vi "Configure System.vi"(8 "error in (no error)":errorcluster, 11 "System Configuration":T1) -> (0 "error out":errorcluster, 3 "dup System Configuration":T1)   [LabVIEW 2024]
doc: "Applies system configurations."
uses:
  Controls/Server/System Configuration.ctl
  Controls/Server/Subsystem Configuration.ctl
  <vilib>/lvdsc/NI_DSC.lvlib
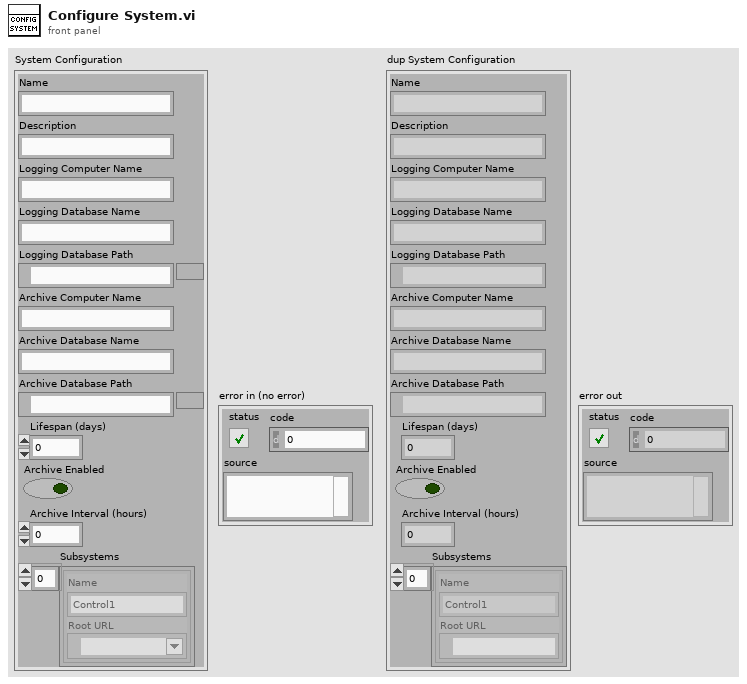
[diagram p1: front panel]
types:
  T1 = typedef "System Configuration.ctl" = cluster{"Name":string, "Description":string, "Logging Computer Name":string, "Logging Database Name":string, "Logging Database Path":path, "Archive Computer Name":string, "Archive Database Name":string, "Archive Database Path":path, "Lifespan (days)":u32, "Archive Enabled":bool, "Archive Interval (hours)":u32, "Subsystems":T2[]}
  T2 = typedef "Subsystem Configuration.ctl" = cluster{"Name":string, "Root URL":refnum<k21>}
  T3 = cluster{"machine":string, "name":string, "path":path}
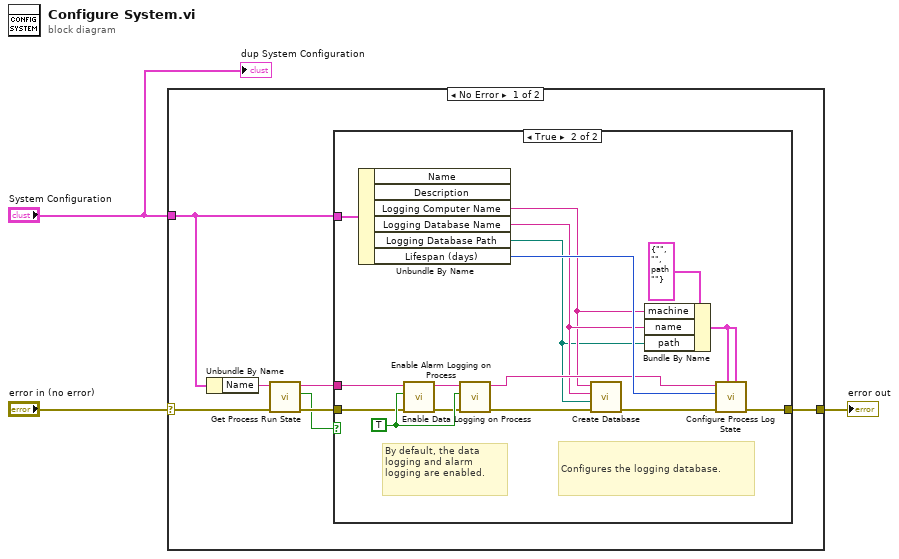
[diagram p0: block diagram]
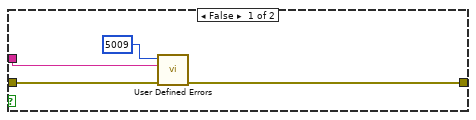
[diagram p2: hidden frame]
diagram:
  n1 = case shown="No Error" "error in (no error)" {
    selector: "error in (no error)" -> [w5 w31]
    tunnel: [w7 w31] -> w3
    tunnel: "System Configuration" -> [w4 _]
    frame No Error {
      n2 = Unbundle By Name(w4) -> ("Name"=w10:string)
      n3 = call <vilib>:"Get Process Run State.vi"("error in (no error)"=w5, "process name"=w10) -> ("error out"=w8:errorcluster, "exists?"=w6:bool, "process name out"=w9:string)  [unwired: 6 in, 1 out]
      n4 = case shown="True" w6 {
        tunnel: w9 -> [w13 w26]
        tunnel: w8 -> [w12 w27]
        tunnel: [w11 w15] -> w7
        tunnel: w4 -> [_ w25]
        frame False {
          n5 = call "User Defined Errors.vi"("error in (no error)"=w12, "Parameter 1"=w13, "Error Code (0)"=5009 ("error code (0)")) -> ("error out"=w11:errorcluster)  [unwired: 8 in]
        }
        frame True {
          w30 = TRUE ("log?")
          # "By default, the data logging and alarm logging are enabled."
          # "Configures the logging database."
          n6 = Unbundle By Name(w25) -> ("Logging Computer Name"=w17:string, "Logging Database Name"=w18:string, "Logging Database Path"=w16:path, "Lifespan (days)"=w22:u32)  [unwired: 2 out]
          n7 = call <vilib>:"Enable Data Logging on Process.vi"("error in (no error)"=w27, "log?"=w30, "process name"=w26) -> ("error out"=w28:errorcluster, "process name out"=w29:string)  [unwired: 7 in]
          n8 = call <vilib>:"Enable Alarm Logging on Process.vi"("error in (no error)"=w28, "log?"=w30, "process name"=w29) -> ("error out"=w21:errorcluster, "process name out"=w19:string)  [unwired: 7 in]
          n9 = call <vilib>:"Create Database.vi"("error in (no error)"=w21, "database path"=w16, "database name"=w18, "computer name"=w17) -> ("error out"=w20:errorcluster)  [unwired: 4 in, 2 out]
          n10 = Bundle By Name(cluster=T3 {"machine"="", "name"="", "path"=path ""} ("data database"), "machine"=w17, "name"=w18, "path"=w16) -> (w23:T3)
          n11 = call <vilib>:"Configure Process Log State.vi"("alarm database"=w23, "data database"=w23, "error in (no error)"=w20, "data lifespan in days (perpetual)"=w22, "process name"=w19) -> ("error out"=w15:errorcluster)  [unwired: 5 in, 1 out]
        }
      }
    }
    frame Error {
    }
  }
  "error out" <- w3
  "dup System Configuration" <- "System Configuration"
